vi "Get Certificate.vi"(8 "Error In":errorcluster, 10 "Password":string="password", 11 "Certificate Path":string="C:\\Users\\20024507\\Desktop\\SSL\\Certificates\\MyServer.pfx") -> (0 "Error Out":errorcluster, 2 "Index Location":i32, 3 "Certificate":refnum<k24>)   [LabVIEW 2014, in "SSL Lib.lvlib"]
doc: "VI Function: This VI opens a reference to the input X.509 certificate and validates the certificate.\n\nVI Version: 1.0\n\nVI Author: Runjhun Agarwal"
uses:
  <userlib>/SSL Library/SSL Lib.lvlib
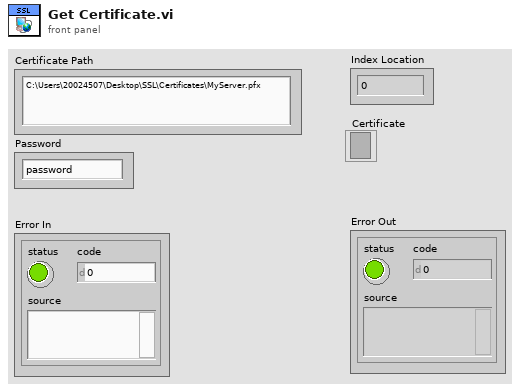
[diagram p1: front panel]
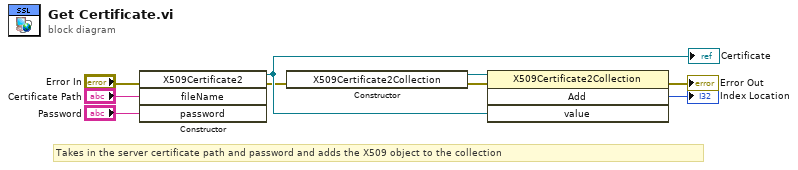
[diagram p0: block diagram]
diagram:
  # "Takes in the server certificate path and password and adds the X509 object to the collection"
  n1 = constructor class="X509Certificate2"(error in="Error In", "fileName"="Certificate Path", "password"="Password") -> (reference out=w7:refnum<k24>, error out=w6:errorcluster)  [unwired: 2 in, 3 out]
  "Certificate" <- w7
  n2 = constructor class="X509Certificate2Collection"(error in=w6) -> (reference out=w4:refnum<k24>, error out=w5:errorcluster)  [unwired: 2 in, 1 out]
  n3 = invoke class="X509Certificate2Collection" method="Add"(reference=w4, error in=w5, "value"=w7) -> (error out=→"Error Out":errorcluster, "Add"=→"Index Location":i32)  [unwired: 1 in, 2 out]
